vi "Data Converter.vi"() -> ()   [LabVIEW 2021]
uses:
  Type Definitions/Data Frame.ctl
  Type Definitions/Data Frame Header.ctl
  Type Definitions/Payload Class.ctl
  Type Definitions/Device.ctl
  Type Definitions/Analog Data.ctl
  Type Definitions/Digital Input Data.ctl
  Type Definitions/Internet Connection Monitor.ctl
  Type Definitions/CPU Usage.ctl
  Type Definitions/Telemetry Recorder Status.ctl
  Type Definitions/Memory Monitor.ctl
  Type Definitions/Queue Monitor.ctl
  Type Definitions/RTOSMonitor.ctl
  Type Definitions/System Time.ctl
panel:
  out "result string 3":string
  out "result string 2":string
  out "result string":string
  out "Numeric 2":i32
  out "error out 3":errorcluster
  out "error out 2":errorcluster
  out "Path":path
  out "appended path":path
  out "Frame":T1 {"CRC" format="%08x"; "Frame Header"."Options" format="%016b"; "Frame Header"."Time" format="%^<%I:%M:%S%3u %p\n%m/%d/%Y %Z>T"; "Frame Header"."Sync" format="%08x"}
  out "Payload ID":u16
  out "Unhandled Data":T1 {"CRC" format="%08x"; "Frame Header"."Options" format="%016b"; "Frame Header"."Time" format="%^<%I:%M:%S%3u %p\n%m/%d/%Y %Z>T"; "Frame Header"."Sync" format="%08x"}
  out "Numeric":i32
  out "error out":errorcluster
  out "data":T1 {"CRC" format="%08x"; "Frame Header"."Options" format="%016b"; "Frame Header"."Time" format="%^<%I:%M:%S%3u %p\n%m/%d/%Y %Z>T"; "Frame Header"."Sync" format="%08x"}
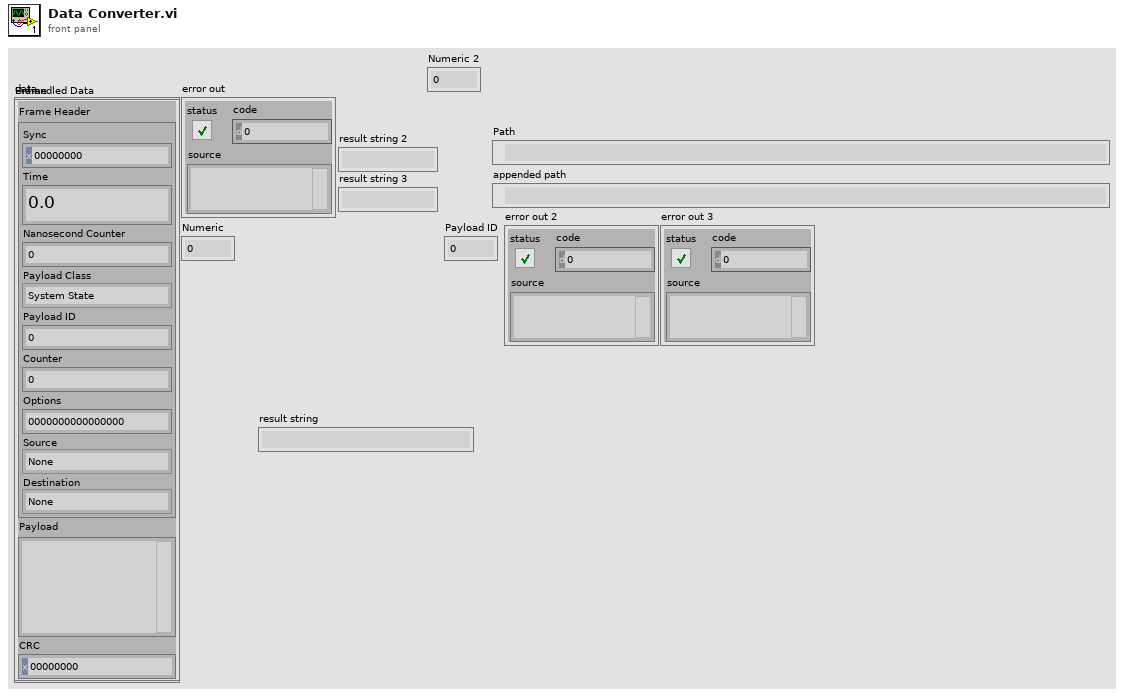
[diagram p1: front panel]
types:
  T1 = typedef "Data Frame.ctl" = cluster{"Frame Header":T2, "Payload":string, "CRC":u32}
  T2 = typedef "Data Frame Header.ctl" = cluster{"Sync":u32, "Time":dbl, "Nanosecond Counter":i64, "Payload Class":T3, "Payload ID":u16, "Counter":i32, "Options":u32, "Source":T4, "Destination":T4}
  T3 = typedef "Payload Class.ctl" = enum16{"System State", "Parameters", "Metadata", "Software Monitor", "Data", "Commands"}
  T4 = typedef "Device.ctl" = enum32{"None", "Exec", "Aux1", "Aux2", "Aux3"}
  T5 = enum16{"open", "open or create", "create or replace", "create", "open (read-only)"}
  T6 = enum16{"open", "replace", "create", "open or create", "replace or create", "replace or create with confirmation"}
  T7 = typedef "Analog Data.ctl" = cluster{"Analog Data":sgl[][]}
  T8 = typedef "Digital Input Data.ctl" = cluster{"Digital Data":u64[][]}
  T9 = typedef "Internet Connection Monitor.ctl" = cluster{"Connected?":bool, "Ping Latency (uS)":i32, "Ping Address":string}
  T10 = typedef "CPU Usage.ctl" = cluster{"User CPU Usage":sgl, "System CPU Usage":sgl, "NIC CPU ":sgl, "IO CPU Usage":sgl, "IRQ CPU Usage":sgl, "SIRQ CPU Usage":sgl, "Idle CPU Time":sgl}
  T11 = typedef "Telemetry Recorder Status.ctl" = cluster{"Filepath":string, "File Size":i64, "Frame Count":i32, "Mean MB/hour":sgl}
  T12 = typedef "Memory Monitor.ctl" = cluster{"Total Memory":sgl, "Available Memory":sgl}
  T13 = typedef "Queue Monitor.ctl" = cluster{"Queue Name":string, "Max Queue Size":i32, "Pending Remove":i32, "Pending Insert":i32, "Elements in Queue":i32}
  T14 = typedef "RTOSMonitor.ctl" = cluster{"Task Name":string, "Priority":i32, "Processor":i32, "Offset":i64, "Min Duration":i64, "Mean Duration":i64, "Max Duration":i64, "Period":i64, "Late Iterations":i16, "Iteration Count":i32}
  T15 = typedef "System Time.ctl" = cluster{"System Clock":timestamp, "GPS Clock":timestamp, "Nanosecond Counter":i64, "GPS Status":enum8{"Initializing", "Normal", "Unable to get fix"}, "GPS Antenna Status":enum8{"Unknown", "Normal", "Absent", "Overcurrent"}, "GPS Satelites Available":u8, "GPS Time (ns)":u64, "GPS UTC Offset":i8, "GPS Time Offset":i32, "UTC Offset Valid":bool, "GPS Time Lock":bool}
  T16 = enum8{"Initializing", "Normal", "Unable to get fix"}
  T17 = enum8{"Unknown", "Normal", "Absent", "Overcurrent"}
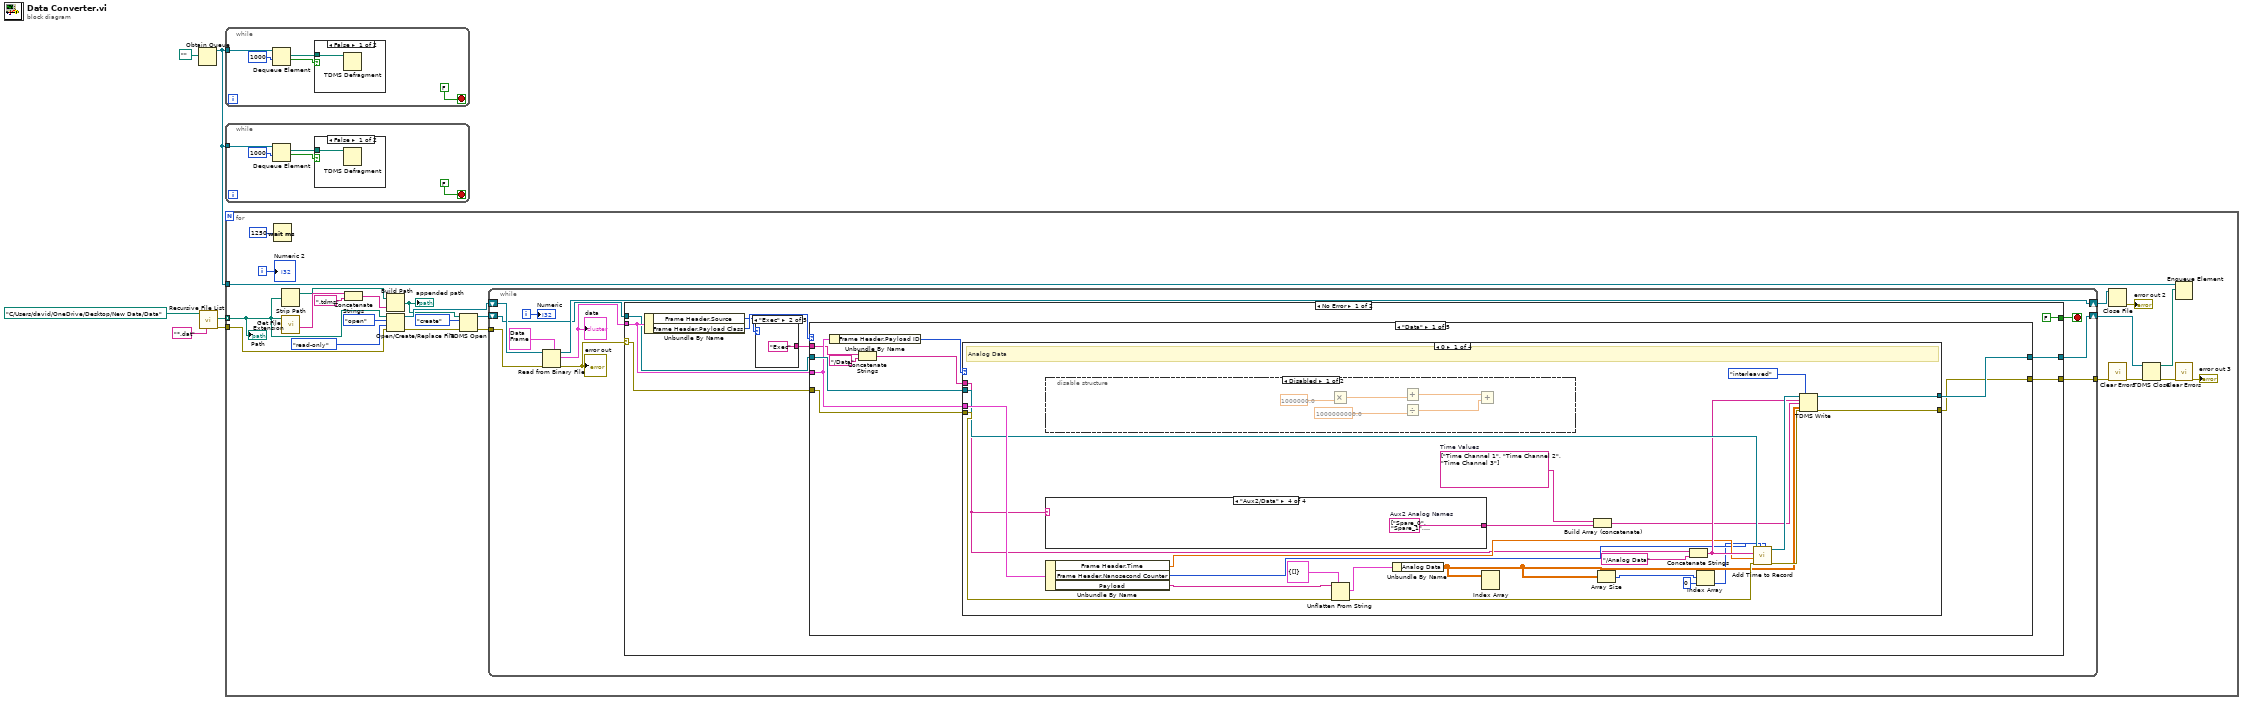
[diagram p0: block diagram]
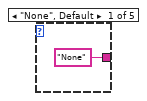
[diagram p4: hidden frame]
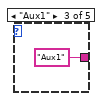
[diagram p5: hidden frame]
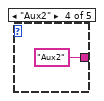
[diagram p6: hidden frame]
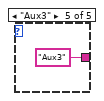
[diagram p7: hidden frame]
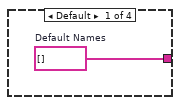
[diagram p8: hidden frame]
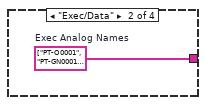
[diagram p9: hidden frame]
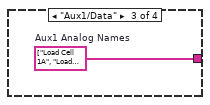
[diagram p10: hidden frame]
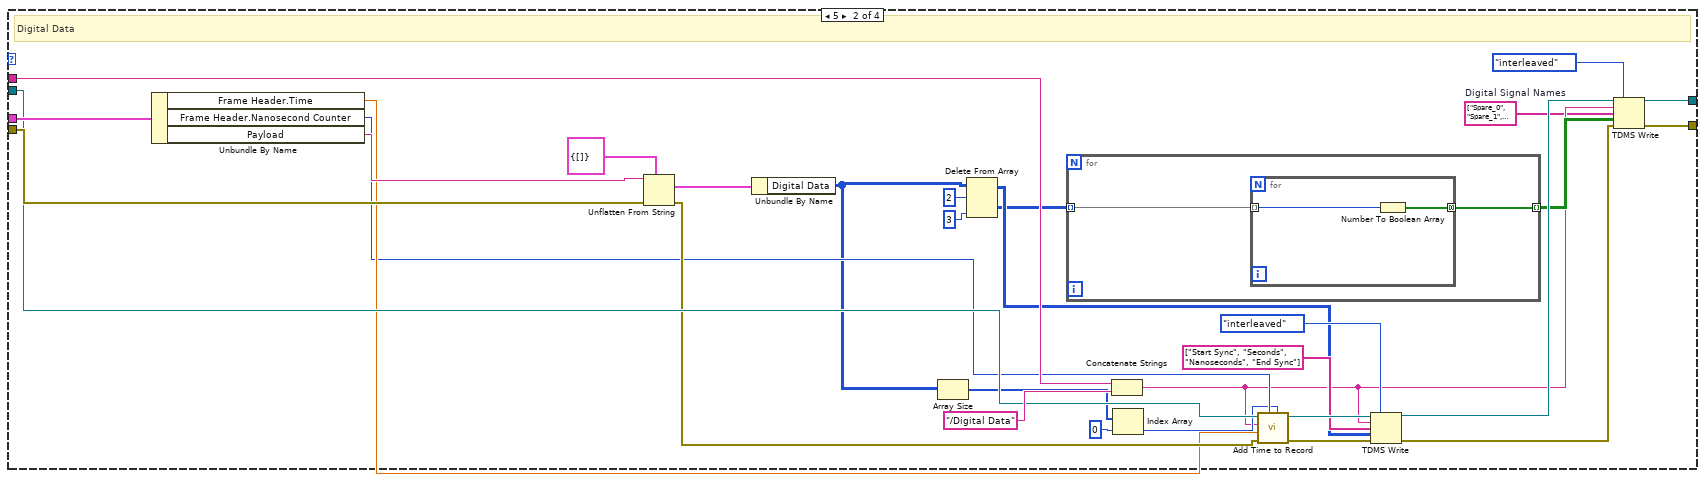
[diagram p12: hidden frame]
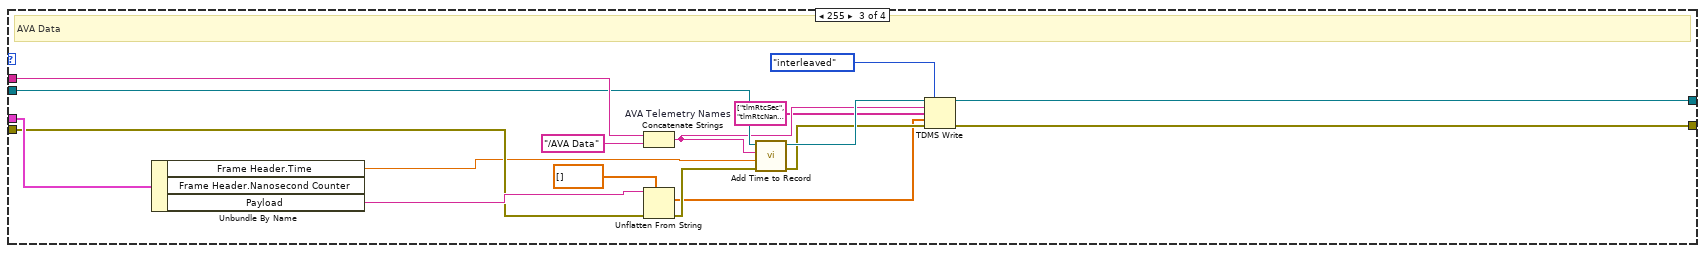
[diagram p13: hidden frame]
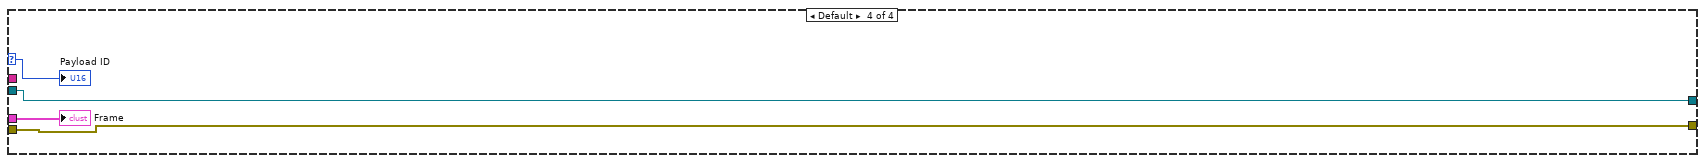
[diagram p14: hidden frame]
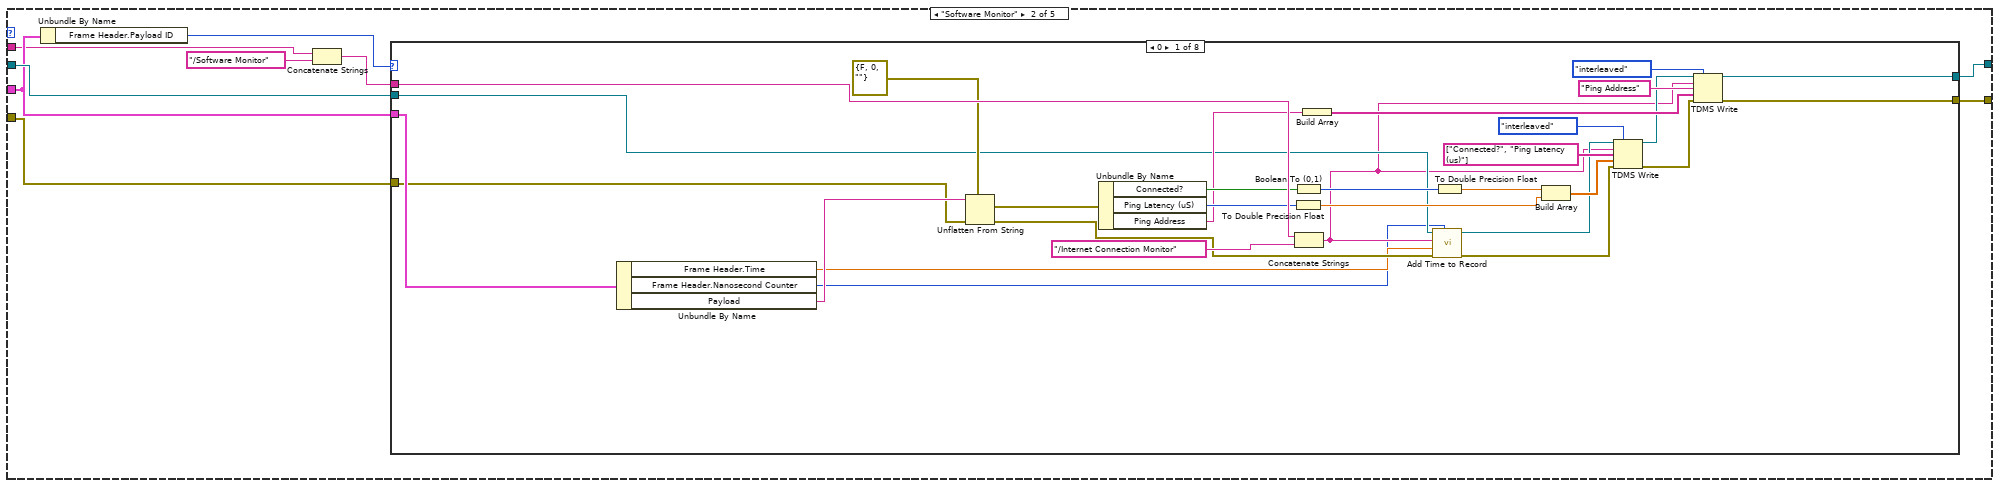
[diagram p15: hidden frame]
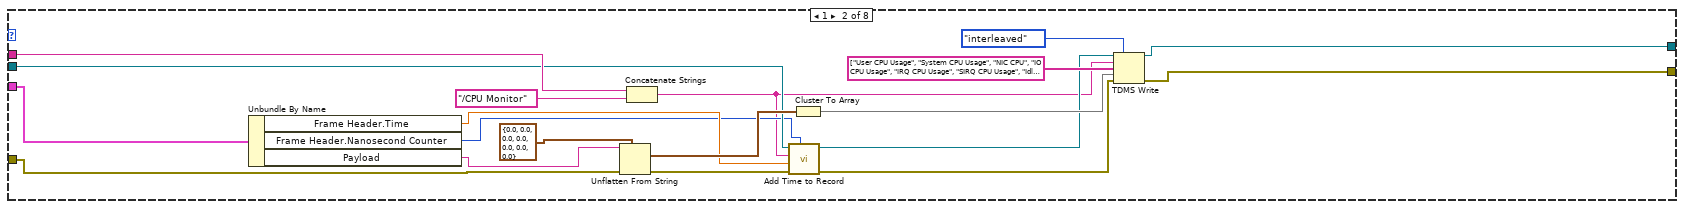
[diagram p16: hidden frame]
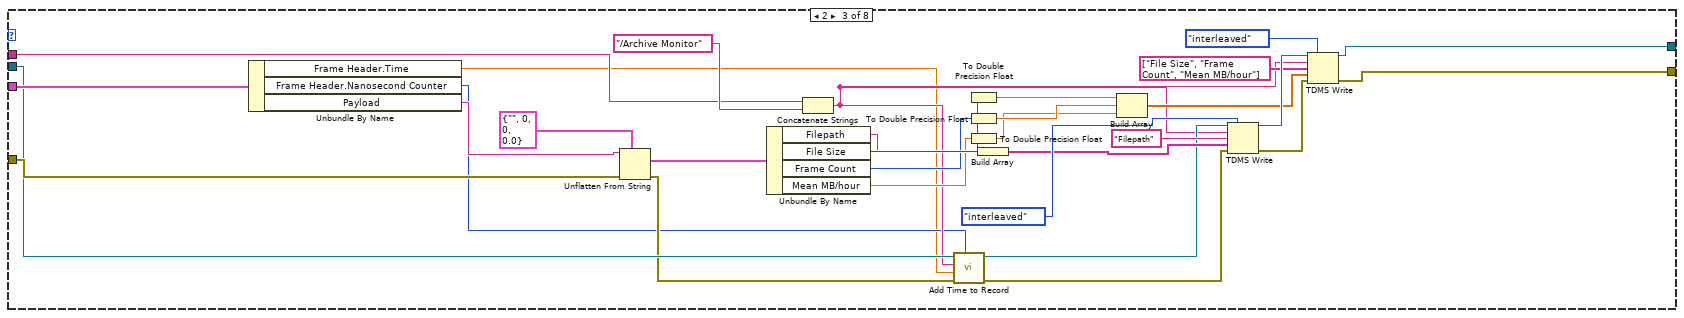
[diagram p17: hidden frame]
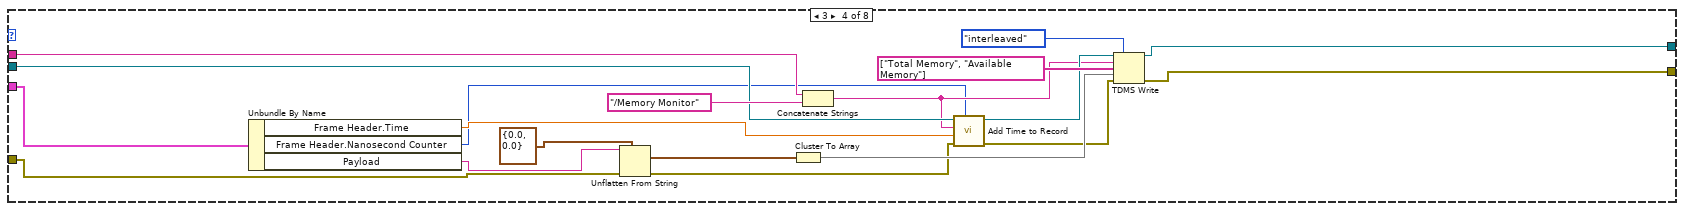
[diagram p18: hidden frame]
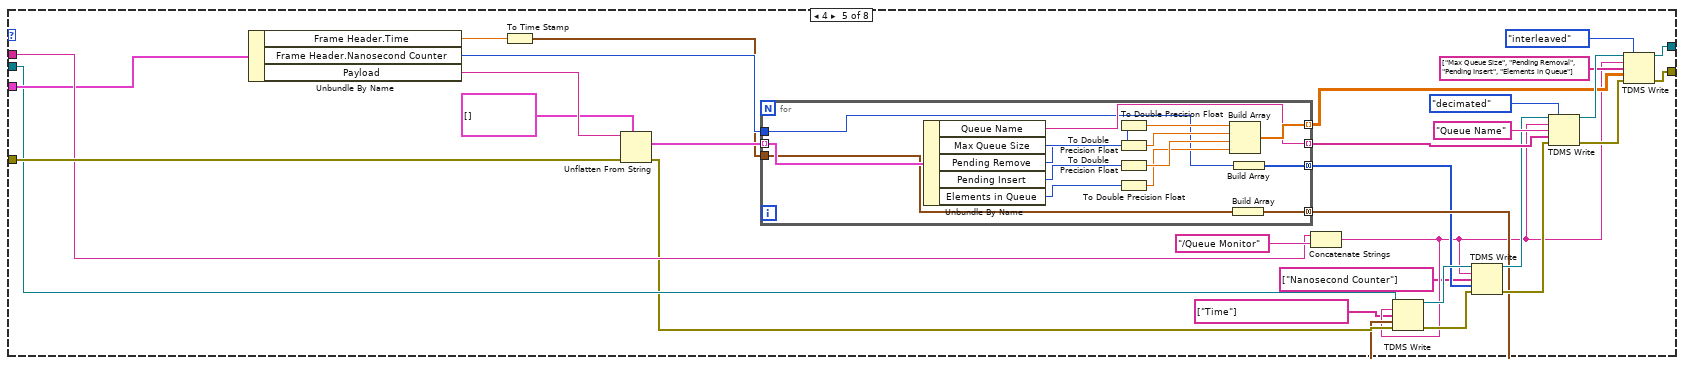
[diagram p19: hidden frame]
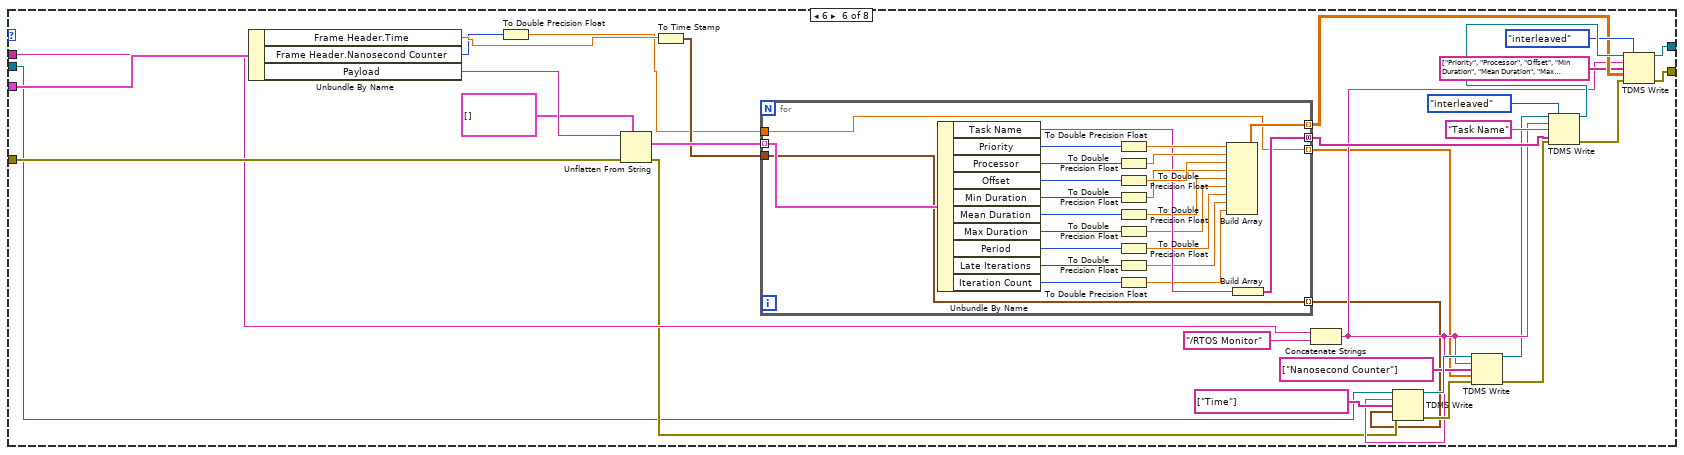
[diagram p20: hidden frame]
diagram:
  n1 = Obtain Queue(element data type=path "" ("file path out")) -> (queue out=w1:refnum<queue>)  [unwired: 4 in, 2 out]
  n2 = call <vilib>:"Recursive File List.vi"("pattern"="*.dat", "Folder Path"=path "C:/Users/david/OneDrive/Desktop/New Data/Data" ("file (use dialog)")) -> ("error out"=w3:errorcluster, "All Files in Dir"=w5:path[])  [unwired: 5 in, 3 out]
  n3 = while {
    tunnel: w1 -> [w11]
    stop <- FALSE stop-if-true
    n4 = Dequeue Element(queue=w11, timeout in ms (-1)=1000) -> (element=w10:path, timed out?=w7:bool)  [unwired: 1 in, 2 out]
    n5 = case shown="False" w7 {
      tunnel: w10 -> [w12 _]
      frame False {
        n6 = TDMS Defragment(7:w12) -> ()  [unwired: 1 in, 1 out]
      }
      frame True {
      }
    }
  }
  n7 = while {
    tunnel: w1 -> [w17]
    stop <- FALSE stop-if-true
    n8 = Dequeue Element(queue=w17, timeout in ms (-1)=1000) -> (element=w16:path, timed out?=w13:bool)  [unwired: 1 in, 2 out]
    n9 = case shown="False" w13 {
      tunnel: w16 -> [w18 _]
      frame False {
        n10 = TDMS Defragment(7:w18) -> ()  [unwired: 1 in, 1 out]
      }
      frame True {
      }
    }
  }
  n11 = for {
    tunnel: w5 -> [w39] mode=indexing
    tunnel: w3 -> [w33]
    tunnel: w1 -> [w20]
    i -> [w22]
    n12 = Wait (ms)(milliseconds to wait=u32 1250) -> ()  [unwired: 1 out]
    n13 = Strip Path(path=w39) -> (stripped path=w36:path)  [unwired: 1 out]
    n14 = call <vilib>:"Get File Extension.vi"("file"=w39) -> ("filename without extension"=w38:string)  [unwired: 6 in, 4 out]
    n15 = Concatenate Strings(w38, ".tdms" ("string")) -> (w35:string)
    n16 = Build Path(base path=w36, name or relative path=w35) -> (appended path=w34:path)
    "appended path" <- w34
    n17 = Open/Create/Replace File(file path (use dialog)=w39, error in=w33, operation (0:open)=T6."open", access (0:read/write)=enum16{"read/write", "read-only", "write-only"}."read-only") -> (refnum out=w41:refnum<file>, error out=w32:errorcluster)  [unwired: 2 in, 1 out]
    n18 = TDMS Open(8:w32, 10:T5."create" ("operation (0:open)"), 11:w34) -> (0:w31:errorcluster, 3:w30:refnum<k34>)  [unwired: 4 in]
    n19 = while {
      shift-right: [w52] -> w28
      shift-left: w41 -> [w53]
      tunnel: w31 -> [w47]
      shift-right: [w46] -> w29
      shift-left: w30 -> [w45]
      tunnel: [w44] -> w25
      i -> [w48]
      stop <- w50 stop-if-true
      n20 = Read from Binary File(5:T1 {"Frame Header"={"Sync"=0, "Time"=0.0, "Nanosecond Counter"=0, "Payload Class"=enum."System State", "Payload ID"=0, "Counter"=0, "Options"=0, "Source"=enum."None", "Destination"=enum."None"}, "Payload"="", "CRC"=0} ("Frame"), 8:w47, 11:w53) -> (0:w51:errorcluster, 2:w49:T1, 3:w52:refnum<file>)  [unwired: 3 in, 1 out]
      "data" <- w49
      "error out" <- w51
      n21 = case shown="No Error" w51 {
        selector: w51 -> [w58 w508]
        tunnel: [FALSE w510] -> w50
        tunnel: w49 -> [w59 _]
        tunnel: w45 -> [w57 w509]
        tunnel: [w56 w509] -> w46
        tunnel: [w55 w508] -> w44
        frame No Error {
          n22 = Unbundle By Name(w59) -> ("Frame Header.Source"=w61:T4, "Frame Header.Payload Class"=w62:T3)
          n23 = case shown="\"Exec\"" w61 {
            tunnel: ["None" "Exec" "Aux1" "Aux2" "Aux3"] -> w60
            frame "None", Default {
            }
            frame "Exec" {
            }
            frame "Aux1" {
            }
            frame "Aux2" {
            }
            frame "Aux3" {
            }
          }
          n24 = case shown="\"Data\"" w62 {
            tunnel: w59 -> [w75 w170 w384 w446 w499]
            tunnel: w57 -> [w76 w174 w388 w450 w503]
            tunnel: [w70 w173 w387 w449 w502] -> w56
            tunnel: [w69 w172 w386 w448 w501] -> w55
            tunnel: w58 -> [w71 w171 w385 w447 w500]
            tunnel: w60 -> [w73 w168 w382 w445 w498]
            frame "Data" {
              n25 = Unbundle By Name(w75) -> ("Frame Header.Payload ID"=w77:u16)
              n26 = Concatenate Strings(w73, "/Data" ("string")) -> (w72:string)
              n27 = case shown="0" w77 {
                selector: w77 -> [_ _ _ w164]
                tunnel: w76 -> [w89 w133 w154 w166]
                tunnel: [w101 w113 w162 w166] -> w70
                tunnel: [w95 w114 w158 w165] -> w69
                tunnel: w71 -> [w98 w139 w159 w165]
                tunnel: w75 -> [w100 w141 w161 w163]
                tunnel: w72 -> [w81 w135 w156 _]
                frame 0 {
                  w80 = string[] ["Time Channel 1", "Time Channel 2", "Time Channel 3"]  # Time Values
                  # "Analog Data"
                  n28 = disable-structure shown="Disabled" {
                    frame Disabled {
                      n29 = Multiply(y=1000000.0) -> (x*y=w109:dbl)  [unwired: 1 in]
                      n30 = Add(y=w109) -> (x+y=w106:dbl)  [unwired: 1 in]
                      n31 = Divide(y=1000000000.0) -> (x/y=w107:dbl)  [unwired: 1 in]
                      n32 = Add(x=w106, y=w107) -> ()  [unwired: 1 out]
                    }
                    frame Enabled {
                    }
                  }
                  n33 = case shown="\"Aux2/Data\"" w81 {
                    tunnel: [w102 w103 w104 w105] -> w79
                    frame Default {
                      w102 = string[] []  # Default Names
                    }
                    frame "Exec/Data" {
                      w103 = string[] ["PT-O0001", "PT-GN0001", "Spare_0", "Spare_1", "Spare_2", "Spare_3", "Spare_4", "Spare_5", "Spare_6", "Spare_7", "Spare_8", "Spare_9", "Spare_10", "Spare_11", "Spare_12", "Spare_13", "HAOP", "HAFP", "Spare_14", "Spare_15", "Spare_16", "Spare_17", "Spare_18", "Spare_19", "Spare_20", "Spare_21", "Spare_22", "Spare_23", "Spare_24", "Spare_25", "Spare_26", "Spare_27"]  # Exec Analog Names
                    }
                    frame "Aux1/Data" {
                      w104 = string[] ["Load Cell 1A", "Load Cell 1B", "Load Cell 2A", "Load Cell 2B", "Load Cell 3A", "Load Cell 3B", "Spare_0", "Spare_1", "Spare_2", "Spare_3", "Spare_4", "Spare_5", "Spare_6", "Spare_7", "Spare_8", "Spare_9", "Spare_10", "Spare_11", "Spare_12", "Spare_13", "Spare_14", "Spare_15", "Spare_16", "Spare_17", "Spare_18", "Spare_19", "Spare_20", "Spare_21", "Spare_22", "Spare_23", "Spare_24", "Spare_25", "Spare_26", "Spare_27", "Spare_28", "Spare_29", "Spare_30", "Spare_31", "Spare_32", "Spare_33", "Spare_34", "Spare_35", "Spare_36", "Spare_37"]  # Aux1 Analog Names
                    }
                    frame "Aux2/Data" {
                      w105 = string[] ["Spare_0", "Spare_1", "Spare_2", "Spare_3", "Spare_4", "Spare_5", "Spare_6", "Spare_7", "Spare_8", "Spare_9", "Spare_10", "Spare_11", "Spare_12", "Spare_13", "Spare_14", "Spare_15", "Spare_16", "Spare_17", "Spare_18", "Spare_19", "Spare_20", "Spare_21", "Spare_22", "Spare_23", "TCX-01", "TCX-02", "TCX-03", "TCX-04", "TCX-05", "TCX-06", "Spare_24", "TCX-07", "Module 4 CJC0", "Module 4 CJC1", "TCX-08", "TCX-09", "TCX-10", "TCX-11", "TCX-12", "TCX-13", "Spare_25", "TCX-14", "Module 5 CJC0", "Module 5 CJC1", "TCX-15", "TCX-16", "TCX-17", "TCX-18", "TCX-19", "TCX-20", "Spare_26", "TCX-21", "Module 6 CJC0", "Module 6 CJC1", "Spare_27", "Spare_28", "Spare_29", "Spare_30"]  # Aux2 Analog Names
                    }
                  }
                  n34 = Unbundle By Name(w100) -> ("Frame Header.Time"=w87:dbl, "Frame Header.Nanosecond Counter"=w86:i64, "Payload"=w99:string)
                  n35 = Unflatten From String(type=T7 {"Analog Data"=[]} ("Analog Data"), binary string=w99, error in (no error)=w98) -> (value=w96:T7, error out=w92:errorcluster)  [unwired: 2 in, 1 out]
                  n36 = Unbundle By Name(w96) -> ("Analog Data"=w85:sgl[][])
                  n37 = Index Array(array=w85) -> ()  [unwired: 2 in, 1 out]
                  n38 = Build Array (concatenate)(w80, w79) -> (w78:string[])
                  n39 = Array Size(array=w85) -> (size(s)=w84:i32[])
                  n40 = Concatenate Strings(w81, "/Analog Data" ("string")) -> (w88:string)
                  n41 = Index Array(array=w84, index=0) -> (element=w82:i32)
                  n42 = call "Add Time to Record.vi"("Array Size (1)"=w82, "Nanosecond Counter"=w86, "error in (no error)"=w92, "Time"=w87, "Group Name"=w88, "TDMS In"=w89) -> ("error out"=w91:errorcluster, "TDMS Out"=w90:refnum<k34>)  [unwired: 4 in]
                  n43 = TDMS Write(0:w90, 1:enum16{"decimated", "interleaved"}."interleaved" ("data layout (0:decimated)"), 5:w88, 7:w78, 9:w85, 11:w91) -> (4:w101:refnum<k34>, 15:w95:errorcluster)  [unwired: 2 out]
                }
                frame 5 {
                  w111 = string[] ["Spare_0", "Spare_1", "Spare_2", "Spare_3", "Spare_4", "Spare_5", "Spare_6", "Spare_7", "Spare_8", "Spare_9", "Spare_10", "Spare_11", "Spare_12", "Spare_13", "Spare_14", "Spare_15", "ROV-G0001_TLKBK CLOSED", "ROV-O0004_TLKBK CLOSED", "ROV-F0002_TLKBK CLOSED", "ROV-F0001_TLKBK CLOSED", "ROV-GN0002_TLKBK CLOSED", "ROV-GN0001_TLKBK CLOSED", "ROV-O0002_TLKBK CLOSED", "ROV-O0001_TLKBK CLOSED", "ROV-G0001_TLKBK OPENED", "ROV-O0004_TLKBK OPENED", "ROV-F0002_TLKBK OPENED", "ROV-F0001_TLKBK OPENED", "ROV-GN0002_TLKBK OPENED", "ROV-GN0001_TLKBK OPENED", "ROV-O0002_TLKBK OPENED", "ROV-O0001_TLKBK OPENED", "Spare_16", "Spare_17", "Spare_18", "Spare_19", "Spare_20", "Spare_21", "Spare_22", "Spare_23", "Spare_24", "Spare_25", "Spare_26", "Spare_27", "Spare_28", "Spare_29", "ROV-N0001_TLKBK CLOSED", "ROV-N0001_TLKBK OPENED", "Spare_30", "Spare_31", "Spare_32", "Spare_33", "Spare_34", "Spare_35", "Spare_36", "Spare_37", "Spare_38", "Spare_39", "Spare_40", "Spare_41", "Spare_42", "Spare_43", "Spare_44", "Spare_45", "OPVV-2", "OPVV-1", "HAFV", "FPVV-2", "FPVV-1", "ROV-N0002", "ROV-N0001", "ROV-G0001", "ROV-O0004", "ROV-A0003", "ROV-F0002", "ROV-F0001", "ROV-GN0002", "ROV-GN0001", "ROV-O0002", "ROV-O0001", "Spare_46", "Spare_47", "Spare_48", "Spare_49", "Spare_50", "Spare_51", "Spare_52", "Spare_53", "Spare_54", "Spare_55", "Spare_56", "Spare_57", "Spare_58", "Spare_59", "Spare_60", "Spare_61", "Spare_62", "Spare_63", "Spare_64", "Spare_65", "Spare_66", "Spare_67", "Spare_68", "Spare_69", "Spare_70", "Spare_71", "Spare_72", "Spare_73", "Spare_74", "Spare_75", "Spare_76", "HAOV", "Spare_77", "Spare_78", "Spare_79", "Spare_80", "Spare_81", "Spare_82", "Spare_83", "Spare_84", "Spare_85", "Spare_86", "Spare_87", "Spare_88", "Spare_89", "Spare_90", "Spare_91", "Spare_92"]  # Digital Signal Names
                  # "Digital Data"
                  n44 = Unbundle By Name(w141) -> ("Frame Header.Time"=w129:dbl, "Frame Header.Nanosecond Counter"=w128:i64, "Payload"=w140:string)
                  n45 = Unflatten From String(type=T8 {"Digital Data"=[]} ("Digital Input Data"), binary string=w140, error in (no error)=w139) -> (value=w138:T8, error out=w130:errorcluster)  [unwired: 2 in, 1 out]
                  n46 = Unbundle By Name(w138) -> ("Digital Data"=w121:u64[][])
                  n47 = Array Size(array=w121) -> (size(s)=w123:i32[])
                  n48 = Delete From Array(array=w121, length=2, index (col)=3 ("disabled index (col)")) -> (deleted portion=w119:u64[][], array with subset deleted=w124:u64[][])  [unwired: 1 in]
                  n49 = for {
                    tunnel: w119 -> [w143] mode=indexing
                    tunnel: [w142] -> w116 mode=indexing
                    n50 = for {
                      tunnel: w143 -> [w145] mode=indexing
                      tunnel: [w144] -> w142 mode=concatenating
                      n51 = Number To Boolean Array(number=w145) -> (Boolean array=w144:bool[])
                    }
                  }
                  n52 = Concatenate Strings(w135, "/Digital Data" ("string")) -> (w115:string)
                  n53 = Index Array(array=w123, index=0) -> (element=w120:i32)
                  n54 = call "Add Time to Record.vi"("Array Size (1)"=w120, "Nanosecond Counter"=w128, "error in (no error)"=w130, "Time"=w129, "Group Name"=w115, "TDMS In"=w133) -> ("error out"=w131:errorcluster, "TDMS Out"=w132:refnum<k34>)  [unwired: 4 in]
                  n55 = TDMS Write(0:w132, 1:enum16{"decimated", "interleaved"}."interleaved" ("data layout (0:decimated)"), 5:w115, 7:string[] ["Start Sync", "Seconds", "Nanoseconds", "End Sync"] ("channel name(s) in (Untitled)"), 9:w124, 11:w131) -> (4:w118:refnum<k34>, 15:w117:errorcluster)  [unwired: 2 out]
                  n56 = TDMS Write(0:w118, 1:enum16{"decimated", "interleaved"}."interleaved" ("data layout (0:decimated)"), 5:w115, 7:w111, 9:w116, 11:w117) -> (4:w113:refnum<k34>, 15:w114:errorcluster)  [unwired: 2 out]
                }
                frame 255 {
                  w146 = string[] ["tlmRtcSec", "tlmRtcNanoSec", "egseTlmFrames", "packetsRcvd", "packetsSent", "lostPacketErrors", "checksumErrors", "missedPackets", "cmdAccepted", "cmdRejected", "vMajor", "vMinor", "vRevision", "POT-1", "POT-2", "POT-3", "POI", "TOT", "TOI", "PFT-1", "PFT-2", "PFT-3", "PFI", "TFT", "TFI", "LoxInletPressEst", "FuelInletPressEst", "NPPT", "NPTC", "NFPT", "NFTC", "OBBPV-1_Cmd", "OBBPV-2_Cmd", "FBBPV-1_Cmd", "FBBPV-2_Cmd", "NVV_Cmd", "NIV_Cmd", "LoxAbortReason", "LoxAbortReasonOverPressure", "LoxAbortReasonVenting", "LoxAbortReasonSensDq", "FuelAbortReason", "FuelAbortReasonOverPressure", "FuelAbortReasonVenting", "FuelAbortReasonSensDq", "FrameCounter", "ClockSeconds", "ClockNanoseconds", "ApplicationState", "SoftwareVersionMajor", "SoftwareVersionMinor", "SoftwareVersionPatch", "LoxTankPressControlActive", "FuelTankPressControlActive", "CommandsAccepted", "CommandsRejected", "Padding_5", "Padding_6", "digitalRedline", "digitalInhibit", "digitalArm", "Padding_7", "ignitionSequenceStatus", "shutdownSequenceStatus", "testSequenceStatus", "CRC"]  # AVA Telemetry Names
                  # "AVA Data"
                  n57 = Unbundle By Name(w161) -> ("Frame Header.Time"=w150:dbl, "Payload"=w160:string)  [unwired: 1 out]
                  n58 = Concatenate Strings(w156, "/AVA Data" ("string")) -> (w149:string)
                  n59 = Unflatten From String(type=dbl[] [], binary string=w160, error in (no error)=w159) -> (value=w147:dbl[], error out=w151:errorcluster)  [unwired: 2 in, 1 out]
                  n60 = call "Add Time to Record.vi"("error in (no error)"=w151, "Time"=w150, "Group Name"=w149, "TDMS In"=w154) -> ("error out"=w152:errorcluster, "TDMS Out"=w153:refnum<k34>)  [unwired: 6 in]
                  n61 = TDMS Write(0:w153, 1:enum16{"decimated", "interleaved"}."interleaved" ("data layout (0:decimated)"), 5:w149, 7:w146, 9:w147, 11:w152) -> (4:w162:refnum<k34>, 15:w158:errorcluster)  [unwired: 2 out]
                }
                frame Default {
                  "Payload ID" <- w164
                  "Frame" <- w163
                }
              }
            }
            frame "Software Monitor" {
              n62 = Unbundle By Name(w170) -> ("Frame Header.Payload ID"=w175:u16)
              n63 = Concatenate Strings(w168, "/Software Monitor" ("string")) -> (w167:string)
              n64 = case shown="0" w175 {
                tunnel: w174 -> [w182 w210 w231 w262 w288 w328 w378 w380]
                tunnel: [w186 w224 w237 w267 w294 w341 w378 w380] -> w173
                tunnel: [w184 w220 w235 w266 w297 w344 w377 w379] -> w172
                tunnel: w171 -> [w203 w221 w253 w272 w304 w350 w377 w379]
                tunnel: w170 -> [w205 w223 w255 w274 w289 w352 _ _]
                tunnel: w167 -> [w200 w218 w251 w270 w302 w348 _ _]
                frame 0 {
                  n65 = Unbundle By Name(w205) -> ("Frame Header.Time"=w178:dbl, "Frame Header.Nanosecond Counter"=w176:i64, "Payload"=w204:string)
                  n66 = Unflatten From String(type=T9 {"Connected?"=FALSE, "Ping Latency (uS)"=0, "Ping Address"=""} ("Internet Connection Monitor"), binary string=w204, error in (no error)=w203) -> (value=w202:T9, error out=w181:errorcluster)  [unwired: 2 in, 1 out]
                  n67 = Unbundle By Name(w202) -> ("Connected?"=w193:bool, "Ping Latency (uS)"=w195:i32, "Ping Address"=w190:string)
                  n68 = Boolean To (0,1)(Boolean=w193) -> (0, 1=w197:i16)
                  n69 = To Double Precision Float(number=w195) -> (double precision float=w194:dbl)
                  n70 = Concatenate Strings(w200, "/Internet Connection Monitor" ("string")) -> (w177:string)
                  n71 = Build Array(w190) -> (w189:string[])
                  n72 = call "Add Time to Record.vi"("Nanosecond Counter"=w176, "error in (no error)"=w181, "Time"=w178, "Group Name"=w177, "TDMS In"=w182) -> ("error out"=w179:errorcluster, "TDMS Out"=w180:refnum<k34>)  [unwired: 5 in]
                  n73 = To Double Precision Float(number=w197) -> (double precision float=w196:dbl)
                  n74 = Build Array(w196, w194) -> (w192:dbl[])
                  n75 = TDMS Write(0:w180, 1:enum16{"decimated", "interleaved"}."interleaved" ("data layout (0:decimated)"), 5:w177, 7:string[] ["Connected?", "Ping Latency (us)"] ("channel name(s) in (Untitled)"), 9:w192, 11:w179) -> (4:w187:refnum<k34>, 15:w185:errorcluster)  [unwired: 2 out]
                  n76 = TDMS Write(0:w187, 1:enum16{"decimated", "interleaved"}."interleaved" ("data layout (0:decimated)"), 5:w177, 7:"Ping Address" ("channel name(s) in (Untitled)"), 9:w189, 11:w185) -> (4:w186:refnum<k34>, 15:w184:errorcluster)  [unwired: 2 out]
                }
                frame 1 {
                  n77 = Unbundle By Name(w223) -> ("Frame Header.Time"=w208:dbl, "Frame Header.Nanosecond Counter"=w207:i64, "Payload"=w222:string)
                  n78 = Unflatten From String(type=T10 {"User CPU Usage"=0.0, "System CPU Usage"=0.0, "NIC CPU "=0.0, "IO CPU Usage"=0.0, "IRQ CPU Usage"=0.0, "SIRQ CPU Usage"=0.0, "Idle CPU Time"=0.0}, binary string=w222, error in (no error)=w221) -> (value=w215:T10, error out=w209:errorcluster)  [unwired: 2 in, 1 out]
                  n79 = Concatenate Strings(w218, "/CPU Monitor" ("string")) -> (w206:string)
                  n80 = call "Add Time to Record.vi"("Nanosecond Counter"=w207, "error in (no error)"=w209, "Time"=w208, "Group Name"=w206, "TDMS In"=w210) -> ("error out"=w211:errorcluster, "TDMS Out"=w212:refnum<k34>)  [unwired: 5 in]
                  n81 = Cluster To Array(cluster=w215) -> (array=w214:sgl[])
                  n82 = TDMS Write(0:w212, 1:enum16{"decimated", "interleaved"}."interleaved" ("data layout (0:decimated)"), 5:w206, 7:string[] ["User CPU Usage", "System CPU Usage", "NIC CPU", "IO CPU Usage", "IRQ CPU Usage", "SIRQ CPU Usage", "Idle CPU Time"] ("channel name(s) in (Untitled)"), 9:w214, 11:w211) -> (4:w224:refnum<k34>, 15:w220:errorcluster)  [unwired: 2 out]
                }
                frame 2 {
                  n83 = Unbundle By Name(w255) -> ("Frame Header.Time"=w225:dbl, "Frame Header.Nanosecond Counter"=w226:i64, "Payload"=w254:string)
                  n84 = Unflatten From String(type=T11 {"Filepath"="", "File Size"=0, "Frame Count"=0, "Mean MB/hour"=0.0}, binary string=w254, error in (no error)=w253) -> (value=w248:T11, error out=w229:errorcluster)  [unwired: 2 in, 1 out]
                  n85 = Unbundle By Name(w248) -> ("Filepath"=w244:string, "File Size"=w247:i64, "Frame Count"=w246:i32, "Mean MB/hour"=w245:sgl)
                  n86 = Concatenate Strings(w251, "/Archive Monitor" ("string")) -> (w227:string)
                  n87 = call "Add Time to Record.vi"("Nanosecond Counter"=w226, "error in (no error)"=w229, "Time"=w225, "Group Name"=w227, "TDMS In"=w231) -> ("error out"=w228:errorcluster, "TDMS Out"=w230:refnum<k34>)  [unwired: 5 in]
                  n88 = To Double Precision Float(number=w247) -> (double precision float=w243:dbl)
                  n89 = To Double Precision Float(number=w246) -> (double precision float=w242:dbl)
                  n90 = To Double Precision Float(number=w245) -> (double precision float=w241:dbl)
                  n91 = Build Array(w244) -> (w240:string[])
                  n92 = Build Array(w243, w242, w241) -> (w233:dbl[])
                  n93 = TDMS Write(0:w230, 1:enum16{"decimated", "interleaved"}."interleaved" ("data layout (0:decimated)"), 5:w227, 7:"Filepath", 9:w240, 11:w228) -> (4:w238:refnum<k34>, 15:w236:errorcluster)  [unwired: 2 out]
                  n94 = TDMS Write(0:w238, 1:enum16{"decimated", "interleaved"}."interleaved" ("data layout (0:decimated)"), 5:w227, 7:string[] ["File Size", "Frame Count", "Mean MB/hour"] ("channel name(s) in (Untitled)"), 9:w233, 11:w236) -> (4:w237:refnum<k34>, 15:w235:errorcluster)  [unwired: 2 out]
                }
                frame 3 {
                  n95 = Unbundle By Name(w274) -> ("Frame Header.Time"=w257:dbl, "Frame Header.Nanosecond Counter"=w256:i64, "Payload"=w273:string)
                  n96 = Unflatten From String(type=T12 {"Total Memory"=0.0, "Available Memory"=0.0}, binary string=w273, error in (no error)=w272) -> (value=w265:T12, error out=w260:errorcluster)  [unwired: 2 in, 1 out]
                  n97 = Cluster To Array(cluster=w265) -> (array=w264:sgl[])
                  n98 = Concatenate Strings(w270, "/Memory Monitor" ("string")) -> (w258:string)
                  n99 = call "Add Time to Record.vi"("Nanosecond Counter"=w256, "error in (no error)"=w260, "Time"=w257, "Group Name"=w258, "TDMS In"=w262) -> ("error out"=w259:errorcluster, "TDMS Out"=w261:refnum<k34>)  [unwired: 5 in]
                  n100 = TDMS Write(0:w261, 1:enum16{"decimated", "interleaved"}."interleaved" ("data layout (0:decimated)"), 5:w258, 7:string[] ["Total Memory", "Available Memory"] ("channel name(s) in (Untitled)"), 9:w264, 11:w259) -> (4:w267:refnum<k34>, 15:w266:errorcluster)  [unwired: 2 out]
                }
                frame 4 {
                  n101 = Unbundle By Name(w289) -> ("Frame Header.Time"=w277:dbl, "Frame Header.Nanosecond Counter"=w280:i64, "Payload"=w305:string)
                  n102 = To Time Stamp(1:w277) -> (0:w276:timestamp)
                  n103 = Unflatten From String(type=T13[] [] ("cluster"), binary string=w305, error in (no error)=w304) -> (value=w299:T13[], error out=w285:errorcluster)  [unwired: 2 in, 1 out]
                  n104 = for {
                    tunnel: w299 -> [w320] mode=indexing
                    tunnel: [w311] -> w293 mode=indexing
                    tunnel: [w310] -> w291 mode=indexing
                    tunnel: [w308] -> w282 mode=concatenating
                    tunnel: w276 -> [w309]
                    tunnel: [w306] -> w281 mode=concatenating
                    tunnel: w280 -> [w307]
                    n105 = Unbundle By Name(w320) -> ("Queue Name"=w310:string, "Max Queue Size"=w319:i32, "Pending Remove"=w318:i32, "Pending Insert"=w317:i32, "Elements in Queue"=w316:i32)
                    n106 = To Double Precision Float(number=w319) -> (double precision float=w315:dbl)
                    n107 = To Double Precision Float(number=w318) -> (double precision float=w314:dbl)
                    n108 = To Double Precision Float(number=w317) -> (double precision float=w313:dbl)
                    n109 = To Double Precision Float(number=w316) -> (double precision float=w312:dbl)
                    n110 = Build Array(w315, w314, w313, w312) -> (w311:dbl[])
                    n111 = Build Array(w309) -> (w308:timestamp[])
                    n112 = Build Array(w307) -> (w306:i64[])
                  }
                  n113 = Concatenate Strings(w302, "/Queue Monitor" ("string")) -> (w279:string)
                  n114 = TDMS Write(0:w288, 5:w279, 7:string[] ["Time"] ("channel name(s) in (Untitled)"), 9:w282, 11:w285) -> (4:w287:refnum<k34>, 15:w284:errorcluster)  [unwired: 1 in, 2 out]
                  n115 = TDMS Write(0:w287, 5:w279, 7:string[] ["Nanosecond Counter"] ("channel name(s) in (Untitled)"), 9:w281, 11:w284) -> (4:w286:refnum<k34>, 15:w283:errorcluster)  [unwired: 1 in, 2 out]
                  n116 = TDMS Write(0:w286, 1:enum16{"decimated", "interleaved"}."decimated" ("data layout (0:decimated)"), 5:w279, 7:"Queue Name", 9:w291, 11:w283) -> (4:w296:refnum<k34>, 15:w298:errorcluster)  [unwired: 2 out]
                  n117 = TDMS Write(0:w296, 1:enum16{"decimated", "interleaved"}."interleaved" ("data layout (0:decimated)"), 5:w279, 7:string[] ["Max Queue Size", "Pending Removal", "Pending Insert", "Elements in Queue"] ("channel name(s) in (Untitled)"), 9:w293, 11:w298) -> (4:w294:refnum<k34>, 15:w297:errorcluster)  [unwired: 2 out]
                }
                frame 6 {
                  n118 = Unbundle By Name(w352) -> ("Frame Header.Time"=w326:dbl, "Frame Header.Nanosecond Counter"=w325:i64, "Payload"=w351:string)
                  n119 = To Double Precision Float(number=w325) -> (double precision float=w321:dbl)
                  n120 = Unflatten From String(type=T14[] [] ("cluster"), binary string=w351, error in (no error)=w350) -> (value=w346:T14[], error out=w330:errorcluster)  [unwired: 2 in, 1 out]
                  n121 = To Time Stamp(1:w326) -> (0:w323:timestamp)
                  n122 = for {
                    tunnel: w346 -> [w376] mode=indexing
                    tunnel: [w367] -> w340 mode=indexing
                    tunnel: [w365] -> w338 mode=concatenating
                    tunnel: [w354] -> w324 mode=indexing
                    tunnel: w323 -> [w354]
                    tunnel: [w353] -> w322 mode=indexing
                    tunnel: w321 -> [w353]
                    n123 = Unbundle By Name(w376) -> ("Task Name"=w366:string, "Priority"=w375:i32, "Processor"=w374:i32, "Offset"=w373:i64, "Min Duration"=w372:i64, "Mean Duration"=w364:i64, "Max Duration"=w363:i64, "Period"=w362:i64, "Late Iterations"=w360:i16, "Iteration Count"=w361:i32)
                    n124 = To Double Precision Float(number=w375) -> (double precision float=w371:dbl)
                    n125 = To Double Precision Float(number=w374) -> (double precision float=w370:dbl)
                    n126 = To Double Precision Float(number=w373) -> (double precision float=w369:dbl)
                    n127 = To Double Precision Float(number=w372) -> (double precision float=w368:dbl)
                    n128 = To Double Precision Float(number=w364) -> (double precision float=w359:dbl)
                    n129 = To Double Precision Float(number=w363) -> (double precision float=w358:dbl)
                    n130 = To Double Precision Float(number=w362) -> (double precision float=w357:dbl)
                    n131 = To Double Precision Float(number=w360) -> (double precision float=w356:dbl)
                    n132 = To Double Precision Float(number=w361) -> (double precision float=w355:dbl)
                    n133 = Build Array(w371, w370, w369, w368, w359, w358, w357, w356, w355) -> (w367:dbl[])
                    n134 = Build Array(w366) -> (w365:string[])
                  }
                  n135 = Concatenate Strings(w348, "/RTOS Monitor" ("string")) -> (w331:string)
                  n136 = TDMS Write(0:w328, 5:w331, 7:string[] ["Time"] ("channel name(s) in (Untitled)"), 9:w324, 11:w330) -> (4:w335:refnum<k34>, 15:w334:errorcluster)  [unwired: 1 in, 2 out]
                  n137 = TDMS Write(0:w335, 5:w331, 7:string[] ["Nanosecond Counter"] ("channel name(s) in (Untitled)"), 9:w322, 11:w334) -> (4:w327:refnum<k34>, 15:w329:errorcluster)  [unwired: 1 in, 2 out]
                  n138 = TDMS Write(0:w327, 1:enum16{"decimated", "interleaved"}."interleaved" ("data layout (0:decimated)"), 5:w331, 7:"Task Name", 9:w338, 11:w329) -> (4:w343:refnum<k34>, 15:w345:errorcluster)  [unwired: 2 out]
                  n139 = TDMS Write(0:w343, 1:enum16{"decimated", "interleaved"}."interleaved" ("data layout (0:decimated)"), 5:w331, 7:string[] ["Priority", "Processor", "Offset", "Min Duration", "Mean Duration", "Max Duration", "Period", "Late Iterations", "Iteration Count"] ("channel name(s) in (Untitled)"), 9:w340, 11:w345) -> (4:w341:refnum<k34>, 15:w344:errorcluster)  [unwired: 2 out]
                }
                frame 5 {
                }
                frame Default {
                }
              }
            }
            frame "Commands" {
              n140 = Unbundle By Name(w384) -> ("Frame Header.Payload ID"=w389:u16)
              n141 = Concatenate Strings(w382, "/Commands" ("string")) -> (w381:string)
              n142 = case shown="2" w389 {
                tunnel: w388 -> [w403 w409 w435]
                tunnel: [w408 w409 w442] -> w387
                tunnel: [w405 w410 w440] -> w386
                tunnel: w385 -> [w406 w410 w431]
                tunnel: w384 -> [w407 _ w441]
                tunnel: w381 -> [w404 _ w438]
                frame 2 {
                  w390 = string[] ["OPVV-2", "OPVV-1", "HAFV", "FPVV-2", "FPVV-1", "ROV-N0002", "ROV-N0001", "ROV-G0001", "ROV-O0004", "ROV-A0003", "ROV-F0002", "ROV-F0001", "ROV-GN0002", "ROV-GN0001", "ROV-O0002", "ROV-O0001", "Spare_46", "Spare_47", "Spare_48", "Spare_49", "Spare_50", "Spare_51", "Spare_52", "Spare_53", "Spare_54", "Spare_55", "Spare_56", "Spare_57", "Spare_58", "Spare_59", "Spare_60", "Spare_61", "Spare_62", "Spare_63", "Spare_64", "Spare_65", "Spare_66", "Spare_67", "Spare_68", "Spare_69", "Spare_70", "Spare_71", "Spare_72", "Spare_73", "Spare_74", "Spare_75", "Spare_76", "HAOV", "Spare_77", "Spare_78", "Spare_79", "Spare_80", "Spare_81", "Spare_82", "Spare_83", "Spare_84", "Spare_85", "Spare_86", "Spare_87", "Spare_88", "Spare_89", "Spare_90", "Spare_91", "Spare_92"]  # Digital Command Names
                  w393 = u64 0  # U64
                  n143 = Unbundle By Name(w407) -> ("Frame Header.Time"=w396:dbl, "Frame Header.Nanosecond Counter"=w395:i64, "Payload"=w402:string)
                  n144 = Unflatten From String(type=w393, binary string=w402, error in (no error)=w406) -> (value=w392:u64, error out=w397:errorcluster)  [unwired: 2 in, 1 out]
                  n145 = Concatenate Strings(w404, "/Digital COmmands" ("string")) -> (w394:string)
                  n146 = call "Add Time to Record.vi"("Nanosecond Counter"=w395, "error in (no error)"=w397, "Time"=w396, "Group Name"=w394, "TDMS In"=w403) -> ("error out"=w398:errorcluster, "TDMS Out"=w399:refnum<k34>)  [unwired: 5 in]
                  n147 = Number To Boolean Array(number=w392) -> (Boolean array=w391:bool[])
                  n148 = TDMS Write(0:w399, 1:enum16{"decimated", "interleaved"}."interleaved" ("data layout (0:decimated)"), 5:w394, 7:w390, 9:w391, 11:w398) -> (4:w408:refnum<k34>, 15:w405:errorcluster)  [unwired: 2 out]
                }
                frame Default {
                }
                frame 254 {
                  n149 = Unbundle By Name(w441) -> ("Frame Header.Time"=w434:dbl, "Frame Header.Nanosecond Counter"=w433:i64, "Payload"=w426:string)
                  n150 = Concatenate Strings(w426) -> (w415:string)
                  n151 = Search and Replace String(replace all?=TRUE ("replace all? (F)"), input string=w415, search string="\u0000", replace string="") -> (result string=w414:string)  [unwired: 4 in, 3 out]
                  n152 = Concatenate Strings(w438, "/AVA Commands" ("string")) -> (w432:string)
                  n153 = call "Add Time to Record.vi"("Nanosecond Counter"=w433, "error in (no error)"=w431, "Time"=w434, "Group Name"=w432, "TDMS In"=w435) -> ("error out"=w436:errorcluster, "TDMS Out"=w437:refnum<k34>)  [unwired: 5 in]
                  n154 = Search and Replace String(replace all?=TRUE ("replace all? (F)"), input string=w414, search string="\r\n", replace string="") -> (result string=w420:string)  [unwired: 4 in, 3 out]
                  n155 = Search and Replace String(replace all?=TRUE ("replace all? (F)"), input string=w420, search string="\n", replace string="") -> (result string=w421:string)  [unwired: 4 in, 3 out]
                  n156 = Search and Replace String(replace all?=TRUE ("replace all? (F)"), input string=w421, search string="\r", replace string="") -> (result string=w416:string)  [unwired: 4 in, 3 out]
                  "result string" <- w416
                  "result string 2" <- w416
                  "result string 3" <- w416
                  n157 = Build Array(w416) -> (w428:string[])
                  n158 = TDMS Write(0:w437, 5:w432, 7:"AVA Commands" ("String"), 9:w428, 11:w436) -> (4:w442:refnum<k34>, 15:w440:errorcluster)  [unwired: 1 in, 2 out]
                }
              }
            }
            frame "System State" {
              n159 = Unbundle By Name(w446) -> ("Frame Header.Payload ID"=w451:u16)
              n160 = Concatenate Strings(w445, "/System State" ("string")) -> (w443:string)
              n161 = case shown="0" w451 {
                tunnel: w450 -> [w493 w495]
                tunnel: [w481 w495] -> w449
                tunnel: [w479 w494] -> w448
                tunnel: w447 -> [w490 w494]
                tunnel: w446 -> [w492 _]
                tunnel: w443 -> [w484 _]
                frame 0 {
                  n162 = Unbundle By Name(w492) -> ("Payload"=w491:string)
                  n163 = Unflatten From String(type=T15 {"System Clock"=timestamp(0 s since 1904-01-01), "GPS Clock"=timestamp(0 s since 1904-01-01), "Nanosecond Counter"=0, "GPS Status"=enum."Initializing", "GPS Antenna Status"=enum."Unknown", "GPS Satelites Available"=0, "GPS Time (ns)"=0, "GPS UTC Offset"=0, "GPS Time Offset"=0, "UTC Offset Valid"=FALSE, "GPS Time Lock"=FALSE}, binary string=w491, error in (no error)=w490) -> (value=w487:T15, error out=w489:errorcluster)  [unwired: 2 in, 1 out]
                  n164 = Unbundle By Name(w487) -> ("System Clock"=w486:timestamp, "GPS Clock"=w485:timestamp, "Nanosecond Counter"=w478:i64, "GPS Status"=w475:T16, "GPS Antenna Status"=w474:T17, "GPS Satelites Available"=w471:u8, "GPS Time (ns)"=w470:u64, "GPS UTC Offset"=w467:i8, "GPS Time Offset"=w466:i32, "UTC Offset Valid"=w462:bool, "GPS Time Lock"=w460:bool)
                  n165 = Build Array(w486, w485) -> (w456:timestamp[])
                  n166 = Boolean To (0,1)(Boolean=w462) -> (0, 1=w464:i16)
                  n167 = Boolean To (0,1)(Boolean=w460) -> (0, 1=w463:i16)
                  n168 = Concatenate Strings(w484, "/System Time" ("string")) -> (w458:string)
                  n169 = To Double Precision Float(number=w467) -> (double precision float=w468:dbl)
                  n170 = To Double Precision Float(number=w466) -> (double precision float=w465:dbl)
                  n171 = TDMS Write(0:w493, 1:enum16{"decimated", "interleaved"}."interleaved" ("data layout (0:decimated)"), 5:w458, 7:string[] ["System Clock", "GPS Clock"] ("channel name(s) in (Untitled)"), 9:w456, 11:w489) -> (4:w482:refnum<k34>, 15:w480:errorcluster)  [unwired: 2 out]
                  n172 = To Double Precision Float(number=w478) -> (double precision float=w477:dbl)
                  n173 = To Double Precision Float(number=w475) -> (double precision float=w476:dbl)
                  n174 = To Double Precision Float(number=w474) -> (double precision float=w473:dbl)
                  n175 = To Double Precision Float(number=w471) -> (double precision float=w472:dbl)
                  n176 = To Double Precision Float(number=w470) -> (double precision float=w469:dbl)
                  n177 = To Double Precision Float(number=w464) -> (double precision float=w461:dbl)
                  n178 = To Double Precision Float(number=w463) -> (double precision float=w454:dbl)
                  n179 = Build Array(w477, w476, w473, w472, w469, w468, w465, w461, w454) -> (w459:dbl[])
                  n180 = TDMS Write(0:w482, 1:enum16{"decimated", "interleaved"}."interleaved" ("data layout (0:decimated)"), 5:w458, 7:string[] ["Nanosecond Counter", "GPS Status", "GPS Antenna Status", "GPS Satelites Available", "GPS Time (ns)", "GPS UTC Offset", "GPS Time Offset", "UTC Offset Valid", "GPS Time Lock"] ("channel name(s) in (Untitled)"), 9:w459, 11:w480) -> (4:w481:refnum<k34>, 15:w479:errorcluster)  [unwired: 2 out]
                }
                frame Default {
                }
              }
            }
            frame Default {
              n181 = Unbundle By Name(w499) -> ("Frame Header.Payload ID"=w504:u16)
              n182 = Concatenate Strings(w498, "/Default" ("string")) -> (w496:string)
              n183 = case shown="Default" w504 {
                tunnel: w503 -> [w507]
                tunnel: [w507] -> w502
                tunnel: [w506] -> w501
                tunnel: w500 -> [w506]
                tunnel: w499 -> [w505]
                tunnel: w496 -> [_]
                frame Default {
                  "Unhandled Data" <- w505
                }
              }
            }
          }
        }
        frame Error {
          n184 = Unbundle By Name(w508) -> ("code"=w511:i32)
          n185 = case shown="0, Default" w511 {
            tunnel: [FALSE TRUE] -> w510
            frame 0, Default {
            }
            frame 4 {
            }
          }
        }
      }
      "Numeric" <- w48
    }
    n186 = Close File(refnum=w28) -> (error out=→"error out 2":errorcluster)  [unwired: 1 in, 1 out]
    n187 = call <vilib>:"Clear Errors.vi"("error in (no error)"=w25) -> ("error out"=w24:errorcluster)  [unwired: 5 in, 1 out]
    n188 = TDMS Close(8:w24, 11:w29) -> (0:w23:errorcluster, 3:w21:path)
    n189 = Enqueue Element(queue=w20, element=w21) -> ()  [unwired: 2 in, 3 out]
    n190 = call <vilib>:"Clear Errors.vi"("error in (no error)"=w23) -> ("error out"=→"error out 3":errorcluster)  [unwired: 5 in, 1 out]
    "Path" <- w39
    "Numeric 2" <- w22
  }
